vi "Search Strings.vi"(10 "Search Strings":string[](array[string]), 11 "Strings to be looked":string[](array[string])) -> (3 "Found?":bool)   [LabVIEW 2016, in "WSsupport.lvlib"]
uses:
  WSsupport.lvlib
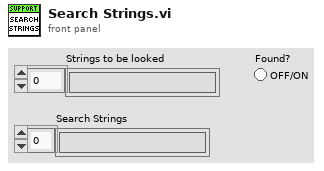
[diagram p1: front panel]
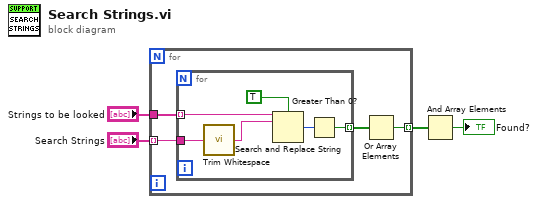
[diagram p0: block diagram]
diagram:
  n1 = for {
    tunnel: "Strings to be looked" -> [w8]
    tunnel: "Search Strings" -> [w7] mode=indexing
    tunnel: [w5] -> w3 mode=indexing
    n2 = for {
      tunnel: w8 -> [w14] mode=indexing
      tunnel: w7 -> [w12]
      tunnel: [w10] -> w6 mode=indexing
      n3 = call <vilib>:"Trim Whitespace.vi"("string"=w12) -> ("trimmed string"=w9:string)  [unwired: 1 in]
      n4 = Search and Replace String(case sensitive?=TRUE ("ignore case? (F)"), input string=w14, search string=w9) -> (number of replacements=w11:i32)  [unwired: 5 in, 3 out]
      n5 = Greater Than 0?(x=w11) -> (x > 0?=w10:bool)
    }
    n6 = Or Array Elements(Boolean array=w6) -> (logical OR=w5:bool)
  }
  n7 = And Array Elements(Boolean array=w3) -> (logical AND=→"Found?":bool)
